vi "VI_bruteforce_salt.vi"(9 "Search space (2^24)":i32=16777216, 11 "Hashes":T1) -> (3 "Salt":string)   [LabVIEW 2023]
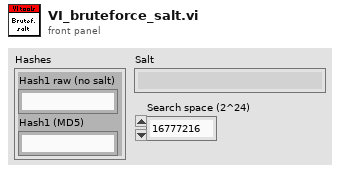
[diagram p1: front panel]
types:
  T1 = cluster{"Hash1 raw (no salt)":string, "Hash1 (MD5)":string}
  T2 = enum16{"big-endian, network order", "native, host order", "little-endian"}
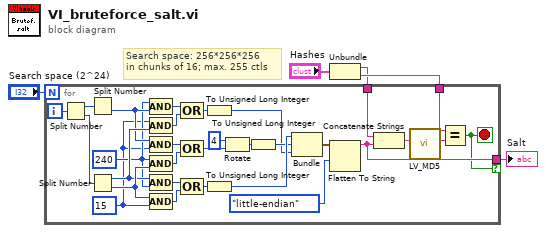
[diagram p0: block diagram]
diagram:
  # "Search space: 256*256*256\nin chunks of 16; max. 255 ctls"
  n1 = Unbundle("Hashes") -> ("Hash1 raw (no salt)"=w1:string, "Hash1 (MD5)"=w2:string)
  n2 = for {
    N: "Search space (2^24)" -> [_]
    tunnel: w1 -> [w12]
    tunnel: w2 -> [w11]
    tunnel: [w10] -> w4 if=w9
    i -> [w8]
    stop <- w9 stop-if-true
    w28 = u8 240
    w27 = u8 15
    n3 = Split Number(x=w8) -> (hi(x)=w35:u16, lo(x)=w34:u16)
    n4 = Split Number(x=w35) -> (lo(x)=w29:u8)  [unwired: 1 out]
    n5 = Split Number(x=w34) -> (hi(x)=w30:u8, lo(x)=w31:u8)
    n6 = Compound Arithmetic op=AND(w28, w29) -> (w23:u8)
    n7 = Compound Arithmetic op=AND(w27, w30) -> (w24:u8)
    n8 = Compound Arithmetic op=AND(w29, w27) -> (w25:u8)
    n9 = Compound Arithmetic op=AND(w28, w31) -> (w26:u8)
    n10 = Compound Arithmetic op=AND(w30, w28) -> (w33:u8)
    n11 = Compound Arithmetic op=AND(w31, w27) -> (w32:u8)
    n12 = Compound Arithmetic op=OR(w23, w24) -> (w18:u8)
    n13 = Compound Arithmetic op=OR(w25, w26) -> (w22:u8)
    n14 = Compound Arithmetic op=OR(w33, w32) -> (w20:u8)
    n15 = To Unsigned Long Integer(number=w18) -> (unsigned 32bit integer=w15:u32)
    n16 = To Unsigned Long Integer(number=w20) -> (unsigned 32bit integer=w17:u32)
    n17 = Rotate(1:w22, 2:i16 4 ("y")) -> (0:w19:u8)
    n18 = To Unsigned Long Integer(number=w19) -> (unsigned 32bit integer=w16:u32)
    n19 = Bundle(w17, w16, w15) -> (w14:cluster{u32, u32, u32})  [unwired: 1 in]
    n20 = Flatten To String(anything=w14, byte order (0:big-endian, network order)=T2."little-endian") -> (data string=w10:string)  [unwired: 2 in, 2 out]
    n21 = Concatenate Strings(w12, w10) -> (w7:string)
    n22 = call "LV_MD5.vi"("Input string"=w7) -> ("MD5 digest (16-bytes)"=w6:string)  [unwired: 9 in, 1 out]
    n23 = Equal?(x=w11, y=w6) -> (x = y?=w9:bool)
  }
  "Salt" <- w4
